vi "Update MSG.vi"(8 "error in (no error)":errorcluster, 10 "Update message":string, 11 "MSG in":refnum<class "MSG.lvclass">) -> (0 "error out":errorcluster, 3 "MSG out":refnum<class "MSG.lvclass">)   [LabVIEW 2020, in "MSG.lvlib" / "MSG.lvclass"]
uses:
  MSG.lvclass
  MSG.lvclass/MSG.ctl
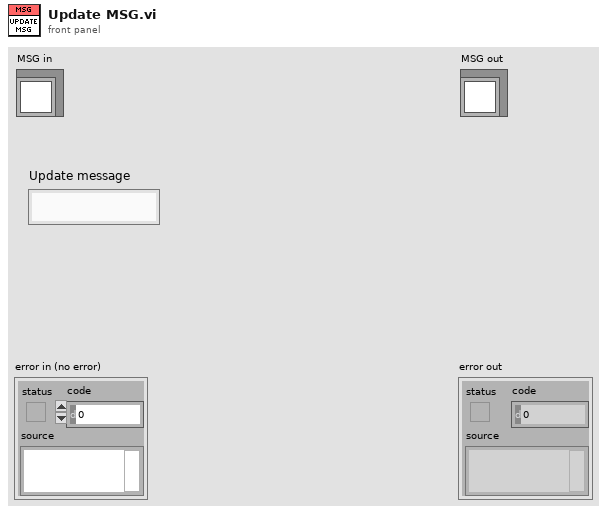
[diagram p1: front panel]
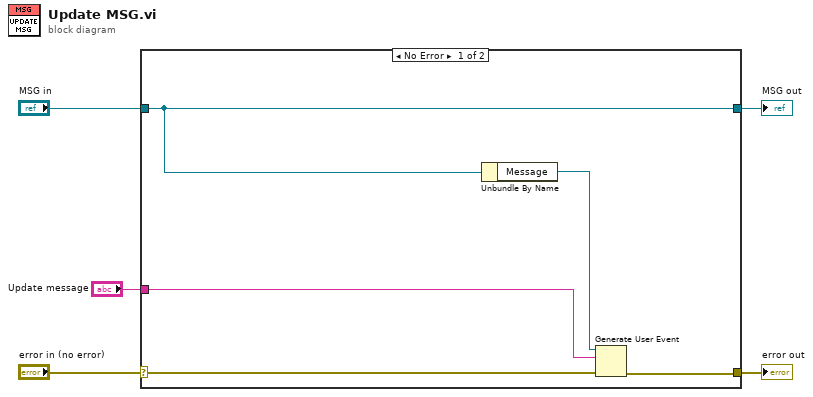
[diagram p0: block diagram]
diagram:
  n1 = case shown="No Error" "error in (no error)" {
    selector: "error in (no error)" -> [w8 w12]
    tunnel: [w9 w12] -> w4
    tunnel: [w10 w11] -> w2
    tunnel: "MSG in" -> [w10 w11]
    tunnel: "Update message" -> [w6 _]
    frame No Error {
      n2 = Unbundle By Name(w10) -> ("Message"=w7:refnum<user-event>)
      n3 = Generate User Event(user event=w7, event data cluster=w6, error in=w8) -> (error out=w9:errorcluster)  [unwired: 1 in, 1 out]
    }
    frame Error {
    }
  }
  "error out" <- w4
  "MSG out" <- w2
